vi "unscaledtoscaledwheader.vi"(1 "array":dbl[](array[numeric]), 2 "Unscaled Data":sgl[](array[numeric])) -> ()   [LabVIEW 2013]
doc: "I. Description:\nThis example reads from the binary file that was created with Acq&Graph to File (Binary).vi. It first reads the header from the file and uses that information to format and scale the data.\n\nII. Instructions for Running:\n1. Browse to your Data File.\n2. Run the VI.\n\nIII. Block Diagram Steps:\n1. Open the file.\n2. Read the first 2 values in the header. Here are the exact contents of the header that were created by Create Header VI: one double for the number of coefficients in the channel, one double for the number of channels in the task, and an array of doubles for the device scaling coefficients (including sample rate).\n3. Given the #coefficients and the #channels we can determine the total size of the header and return that array.\n4. Reshape the 1D array into a 2D array with each channel's information in a separate column \n5. Determine how many bytes remain in the file and read the rest of the information\n6. Call the Convert Unscaled to Scaled Data VI to interpolate the binary data and return the scaled data\n7. Close the file, and check for errors."
panel:
  out "Scaled Data":dbl[](array[numeric])
  # "For instructions, select Help>>Show Context Help"
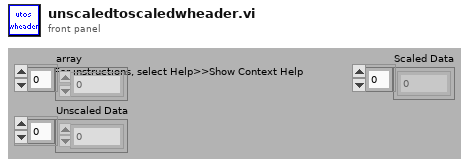
[diagram p1: front panel]
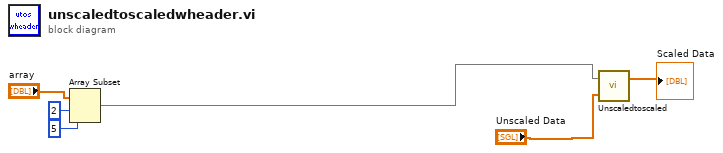
[diagram p0: block diagram]
diagram:
  n1 = Array Subset(array="array", index=2, length=5) -> (w3:dbl[])
  n2 = call "Unscaledtoscaled.vi"("Unscaled Data"="Unscaled Data", "Header Information"=w3) -> ("Array"=→"Scaled Data":dbl[])  [unwired: 1 in]
